vi "datahandleMVL.vi"(0 "xyz array in":dbl[][][](array[numeric]), 1 "action":T1(ring), 5 "Time array in":i32[][](array[numeric]), 7 "error in":errorcluster, 9 "xyz in":dbl[](array[numeric]), 10 "number of frames":i32, 11 "time data in":i32[](array[numeric]), 12 "tracked frame#":i32, 14 "bead number":i32, 15 "number of beads":i32) -> (4 "XYZ out":dbl[][][](array[numeric]), 6 "time out":i32[][](array[numeric]), 8 "error in 2":errorcluster)   [LabVIEW 2011, in "OfflineTracker.lvlib"]
uses:
  OfflineTracker.lvlib
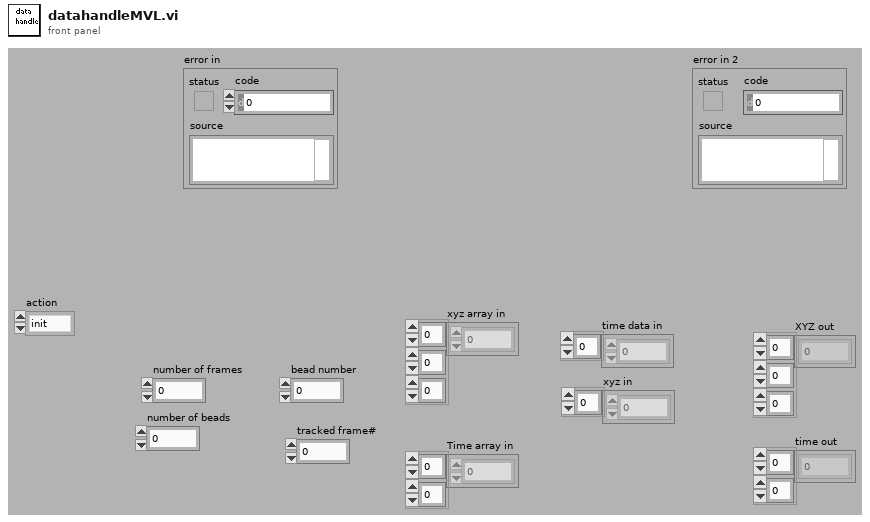
[diagram p1: front panel]
types:
  T1 = enum16{"init", "get", "set single frame", "set all"}
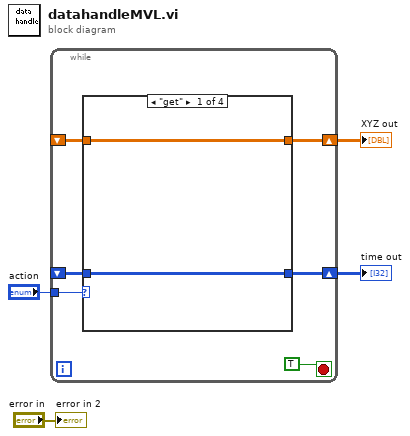
[diagram p0: block diagram]
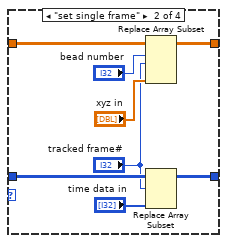
[diagram p2: hidden frame]
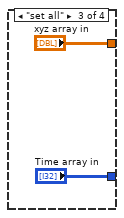
[diagram p3: hidden frame]
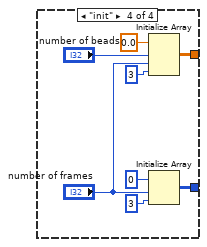
[diagram p4: hidden frame]
diagram:
  n1 = while {
    shift-right: [w8] -> w3
    shift-left: _ -> [w9]
    shift-right: [w7] -> w2
    shift-left: _ -> [w6]
    tunnel: "action" -> [w5]
    stop <- TRUE ("stop") stop-if-true
    n2 = case shown="\"get\"" w5 {
      tunnel: w9 -> [w12 w17 _ _]
      tunnel: [w12 w20 "xyz array in" w30] -> w8
      tunnel: [w11 w15 "Time array in" w23] -> w7
      tunnel: w6 -> [w11 w16 _ _]
      frame "get" {
      }
      frame "set single frame" {
        n3 = Replace Array Subset(array=w17, new element="xyz in", index (dim 0)="bead number", index (dim 1)="tracked frame#") -> (w20:dbl[][][])  [unwired: 1 in]
        n4 = Replace Array Subset(array=w16, new element="time data in", index (row)="tracked frame#") -> (w15:i32[][])  [unwired: 1 in]
      }
      frame "set all" {
      }
      frame "init" {
        n5 = Initialize Array(0.0 ("element"), "number of beads", "number of frames", 3 ("dimension size")) -> (w30:dbl[][][])
        n6 = Initialize Array(0 ("element"), "number of frames", 3 ("dimension size")) -> (w23:i32[][])
      }
    }
  }
  "XYZ out" <- w3
  "time out" <- w2
  "error in 2" <- "error in"
